vi "UpdateSelectedProperty.vi"(8 "error in (no error)":errorcluster, 11 "MetaDriver_v1 in":refnum<class "MetaDriver_v1.lvclass">) -> (0 "error out":errorcluster, 3 "MetaDriver_v1 out":refnum<class "MetaDriver_v1.lvclass">)   [LabVIEW 2020, in "MetaDriver_v1.lvclass"]
doc: "Update the value of the SelectedProperty in the Settings cluster"
uses:
  MetaDriver_v1.lvclass
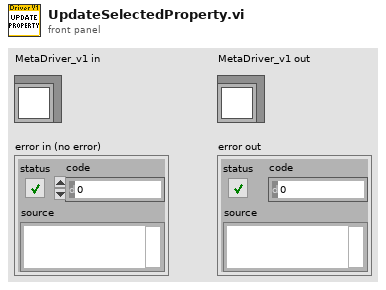
[diagram p1: front panel]
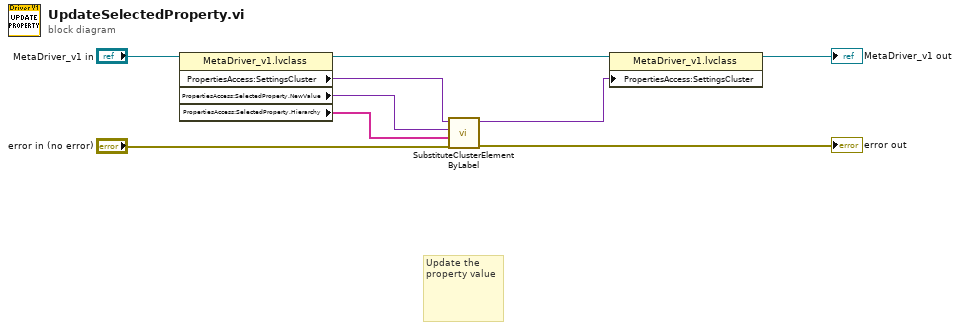
[diagram p0: block diagram]
diagram:
  # "Update the property value"
  n1 = property class="MetaDriver_v1.lvclass"(reference="MetaDriver_v1 in") -> (reference out=w6:refnum<class "MetaDriver_v1.lvclass">, "PropertiesAccess:SettingsCluster"=w2:variant, "PropertiesAccess:SelectedProperty.NewValue"=w7:variant, "PropertiesAccess:SelectedProperty.Hierarchy"=w8:string[])  [unwired: 1 in, 1 out]
  n2 = call "SubstituteClusterElementByLabel.vi"("error in (no error)"="error in (no error)", "ElementHierarchy"=w8, "NewElementValue"=w7, "ClusterIn"=w2) -> ("ErrorOut"=→"error out":errorcluster, "UpdatedClusterOut"=w1:variant)  [unwired: 5 in, 1 out]
  n3 = property class="MetaDriver_v1.lvclass"(reference=w6, "PropertiesAccess:SettingsCluster"=w1) -> (reference out=→"MetaDriver_v1 out":refnum<class "MetaDriver_v1.lvclass">)  [unwired: 1 in, 1 out]
